vi "AVS_GetVersionInfo.vi"(0 "a_hDevice":i32, 7 "a_pFPGAVersion":i8[](array[numeric]), 9 "a_pFirmwareVersion":i8[](array[numeric]), 11 "a_pDLLVersion":i8[](array[numeric])) -> (4 "Output Value":i32, 8 "a_pFPGAVersion":i8[](array[numeric]), 10 "a_pFirmwareVersion":i8[](array[numeric]), 15 "a_pDLLVersion":i8[](array[numeric]))   [LabVIEW 2016]
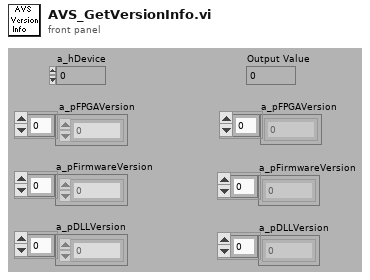
[diagram p1: front panel]
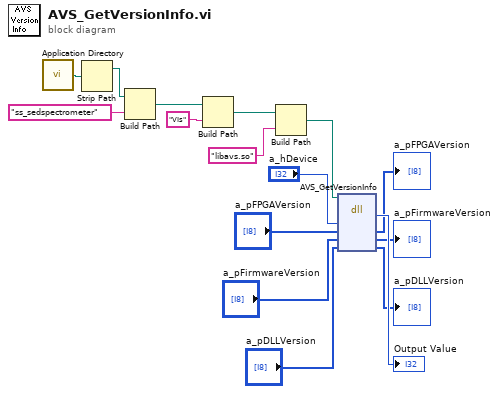
[diagram p0: block diagram]
diagram:
  n1 = call <vilib>:"Application Directory.vi"() -> ("Application Directory"=w5:path)
  n2 = Strip Path(path=w5) -> (stripped path=w4:path)  [unwired: 1 out]
  n3 = Build Path(base path=w4, name or relative path="ss_sedspectrometer") -> (appended path=w7:path)
  n4 = Build Path(base path=w7, name or relative path="VIs") -> (appended path=w2:path)
  n5 = Build Path(base path=w2, name or relative path="libavs.so") -> (appended path=w1:path)
  n6 = dll-call lib="home/harini/Documents/lsst-ts/ts_FiberSpectrograph/ss_sedspectrometer/VIs/libavs.so" fn="AVS_GetVersionInfo"(path in=w1, "a_hDevice"="a_hDevice", "a_pFPGAVersion"="a_pFPGAVersion", "a_pFirmwareVersion"="a_pFirmwareVersion", "a_pDLLVersion"="a_pDLLVersion") -> ("return type"=→"Output Value":i32, "a_pFPGAVersion"=→"a_pFPGAVersion":i8[], "a_pFirmwareVersion"=→"a_pFirmwareVersion":i8[], "a_pDLLVersion"=→"a_pDLLVersion":i8[])  [unwired: 3 in, 2 out]
